vi "Write Name.vi"(8 "error in (no error)":errorcluster, 10 "Name":string, 11 "Chat Window Model in":refnum<class "Chat Window Model.lvclass">) -> (0 "error out":errorcluster, 3 "Chat Window Model out":refnum<class "Chat Window Model.lvclass">)   [LabVIEW 2015, in "Chat Window Model.lvlib" / "Chat Window Model.lvclass"]
uses:
  Chat Window Model.lvclass
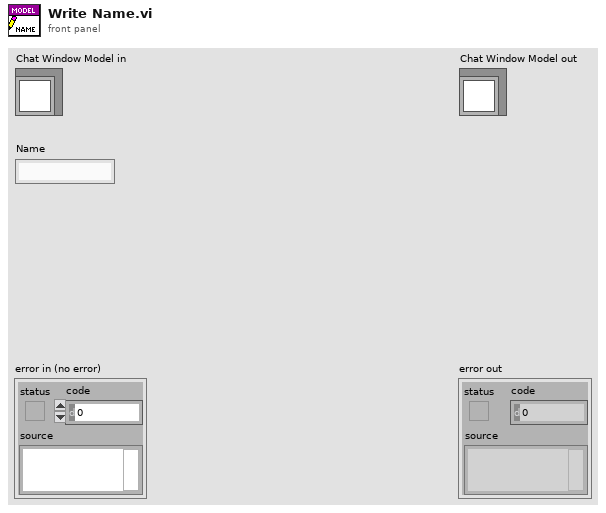
[diagram p1: front panel]
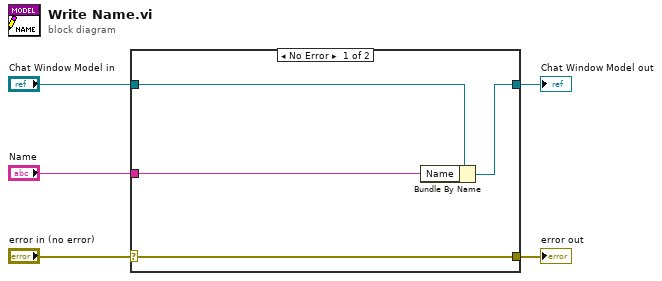
[diagram p0: block diagram]
diagram:
  n1 = case shown="No Error" "error in (no error)" {
    selector: "error in (no error)" -> [w9 w10]
    tunnel: [w9 w10] -> w4
    tunnel: [w6 w11] -> w2
    tunnel: "Chat Window Model in" -> [w8 w11]
    tunnel: "Name" -> [w7 _]
    frame No Error {
      n2 = Bundle By Name(cluster=w8, "Name"=w7) -> (w6:refnum<class "Chat Window Model.lvclass">)
    }
    frame Error {
    }
  }
  "error out" <- w4
  "Chat Window Model out" <- w2
